vi "Initial Data.vi"(8 "error in (no error)":errorcluster, 11 "Master in":refnum<class "Master.lvclass">) -> (0 "error out":errorcluster, 3 "Master out":refnum<class "Master.lvclass">)   [LabVIEW 2014, in "Master.lvclass"]
uses:
  Master/Master.lvclass
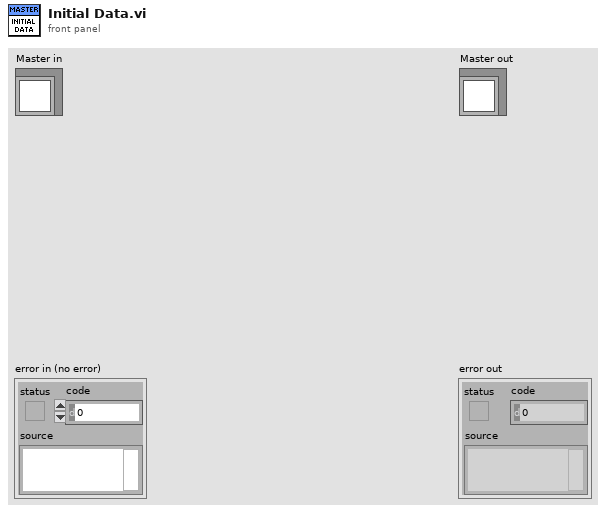
[diagram p1: front panel]
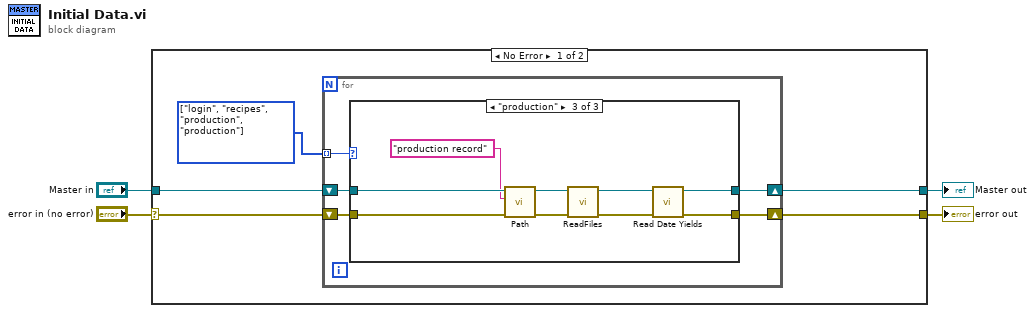
[diagram p0: block diagram]
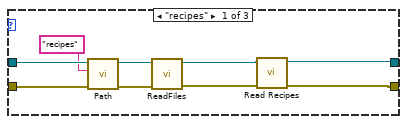
[diagram p2: hidden frame]
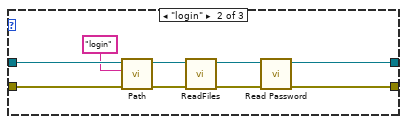
[diagram p3: hidden frame]
diagram:
  n1 = case shown="No Error" "error in (no error)" {
    selector: "error in (no error)" -> [w8 w43]
    tunnel: [w5 w43] -> w3
    tunnel: [w6 w42] -> w1
    tunnel: "Master in" -> [w9 w42]
    frame No Error {
      w7 = enum16{"login", "recipes", "production"}[] [enum."login", enum."recipes", enum."production", enum."production"] items=["login", "recipes", "production"]
      n2 = for {
        shift-right: [w11] -> w6
        shift-left: w9 -> [w14]
        shift-right: [w10] -> w5
        shift-left: w8 -> [w13]
        tunnel: w7 -> [w12] mode=indexing
        n3 = case shown="\"production\"" w12 {
          tunnel: w14 -> [w23 w32 w41]
          tunnel: w13 -> [w22 w31 w40]
          tunnel: [w21 w30 w39] -> w11
          tunnel: [w20 w29 w38] -> w10
          frame "recipes" {
            n4 = call-dynamic "Path.vi"("error in (no error)"=w22, "pathname"="recipes", "Master in"=w23) -> ("error out"=w17:errorcluster, "Master out"=w18:refnum<class "Master.lvclass">)  [unwired: 7 in]
            n5 = call-dynamic "ReadFiles.vi"("error in (no error)"=w17, "Master in"=w18) -> ("error out"=w15:errorcluster, "Master out"=w16:refnum<class "Master.lvclass">)  [unwired: 8 in]
            n6 = call-dynamic "Read Recipes.vi"("error in (no error)"=w15, "Master in"=w16) -> ("error out"=w20:errorcluster, "Master out"=w21:refnum<class "Master.lvclass">)  [unwired: 8 in]
          }
          frame "login" {
            n7 = call-dynamic "Path.vi"("error in (no error)"=w31, "pathname"="login", "Master in"=w32) -> ("error out"=w26:errorcluster, "Master out"=w27:refnum<class "Master.lvclass">)  [unwired: 7 in]
            n8 = call-dynamic "ReadFiles.vi"("error in (no error)"=w26, "Master in"=w27) -> ("error out"=w24:errorcluster, "Master out"=w25:refnum<class "Master.lvclass">)  [unwired: 8 in]
            n9 = call-dynamic "Read Password.vi"("error in (no error)"=w24, "Master in"=w25) -> ("error out"=w29:errorcluster, "Master out"=w30:refnum<class "Master.lvclass">)  [unwired: 8 in]
          }
          frame "production" {
            n10 = call-dynamic "Path.vi"("error in (no error)"=w40, "pathname"="production record", "Master in"=w41) -> ("error out"=w34:errorcluster, "Master out"=w33:refnum<class "Master.lvclass">)  [unwired: 7 in]
            n11 = call-dynamic "ReadFiles.vi"("error in (no error)"=w34, "Master in"=w33) -> ("error out"=w36:errorcluster, "Master out"=w35:refnum<class "Master.lvclass">)  [unwired: 8 in]
            n12 = call-dynamic "Read Date Yields.vi"("error in (no error)"=w36, "Master in"=w35) -> ("error out"=w38:errorcluster, "Master out"=w39:refnum<class "Master.lvclass">)  [unwired: 8 in]
          }
        }
      }
    }
    frame Error {
    }
  }
  "error out" <- w3
  "Master out" <- w1
